vi "Cluster Info.vi"(8 "error in (no error)":errorcluster, 11 "Cluster Variant":variant) -> (0 "error out":errorcluster, 1 "Name":string, 2 "Treat As Array":bool, 3 "Cluster Elements":variant[](array[variant]))   [LabVIEW 2019, in "JKI JSON Serialization.lvlib" / "JSON Serializer.lvclass"]
doc: "JKI JSON 1.1.10.37\nTomi Maila - JKI\nCopyright (c) 2017, JKI"
uses:
  JSON Serializer.lvclass
  <vilib>/Utility/VariantDataType/VariantType.lvlib
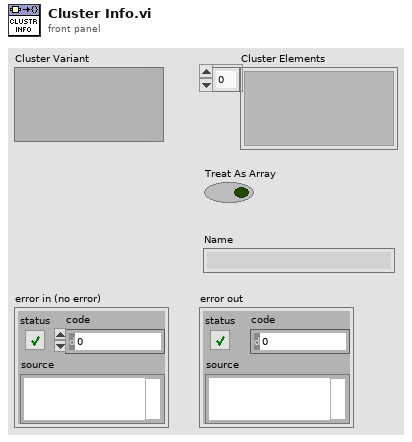
[diagram p1: front panel]
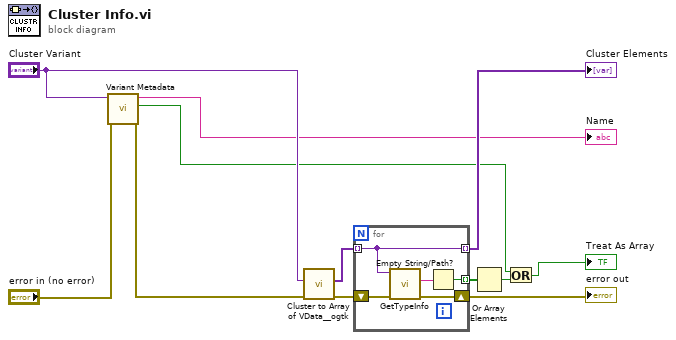
[diagram p0: block diagram]
diagram:
  n1 = call "Variant Metadata.vi"("error in (no error)"="error in (no error)", "Variant"="Cluster Variant") -> ("error out"=w5:errorcluster, "Treat As Array"=w1:bool, "Name"=→"Name":string)  [unwired: 7 in]
  n2 = call "Cluster to Array of VData__ogtk.vi"("error in (no error)"=w5, "Cluster"="Cluster Variant") -> ("error out"=w8:errorcluster, "Array of VData"=w9:variant[])  [unwired: 8 in]
  n3 = for {
    shift-right: [w15] -> w10
    shift-left: w8 -> [w17]
    tunnel: w9 -> [w16] mode=indexing
    tunnel: [w16] -> w11 mode=indexing
    tunnel: [w13] -> w12 mode=indexing
    n4 = call <vilib>:"GetTypeInfo.vi"("error in (no error)"=w17, "Variant"=w16) -> ("error out"=w15:errorcluster, "Name"=w14:string)  [unwired: 5 in, 3 out]
    n5 = Empty String/Path?(string/path=w14) -> (empty?=w13:bool)
  }
  "Cluster Elements" <- w11
  "error out" <- w10
  n6 = Or Array Elements(Boolean array=w12) -> (logical OR=w4:bool)
  n7 = Or(x=w1, y=w4) -> (x .or. y?=→"Treat As Array":bool)
